vi "LINC Insert Data.vi"(0 "item names":string[](array[string]), 1 "member types":string[](array[string]), 2 "scale":bool, 3 "simulate":bool, 5 "item formats":T1[](array[typedef]), 7 "data in":string, 9 "little endian":bool, 11 "error in (no error)":errorcluster, 12 "member names":string[](array[string]), 13 "member data":string[](array[string])) -> (8 "data out":string, 15 "error out":errorcluster)   [LabVIEW 2018, in "STEPkgDriver_LINC.lvlib"]
uses:
  STEPkgDriver_LINC.lvlib
  LINC Format Prototype.ctl
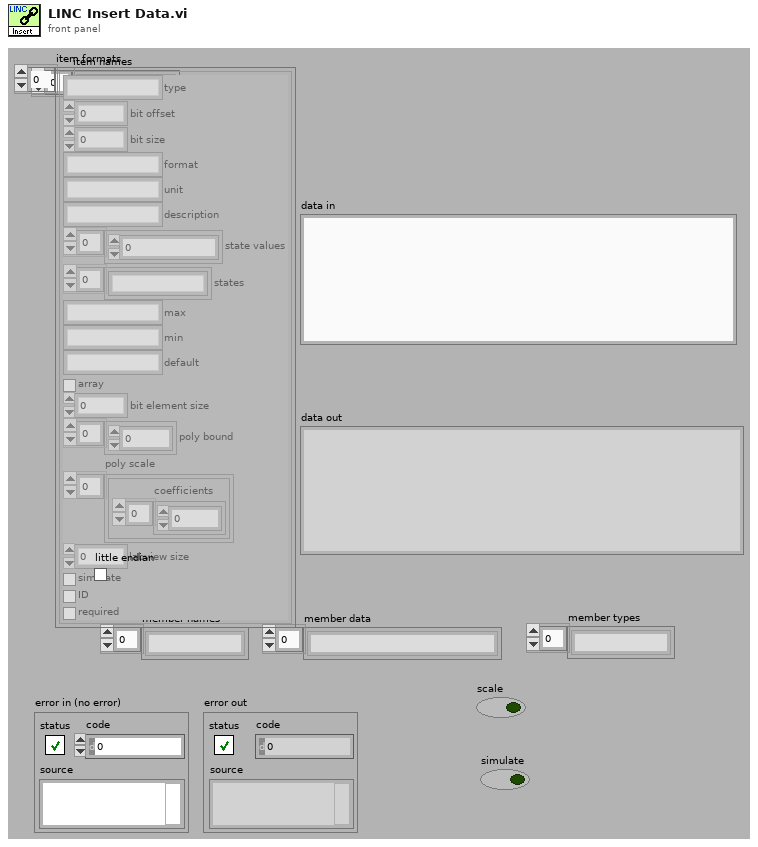
[diagram p1: front panel]
types:
  T1 = typedef "STEPkgDriver_LINC.lvlib/LINC Format Prototype.ctl" = cluster{"type":string, "bit offset":i32, "bit size":i32, "format":string, "unit":string, "description":string, "state values":i64[], "states":string[], "max":string, "min":string, "default":string, "array":bool, "bit element size":i32, "poly bound":dbl[], "poly scale":cluster{"coefficients":dbl[]}[], "labview size":i32, "simulate":bool, "ID":bool, "required":bool}
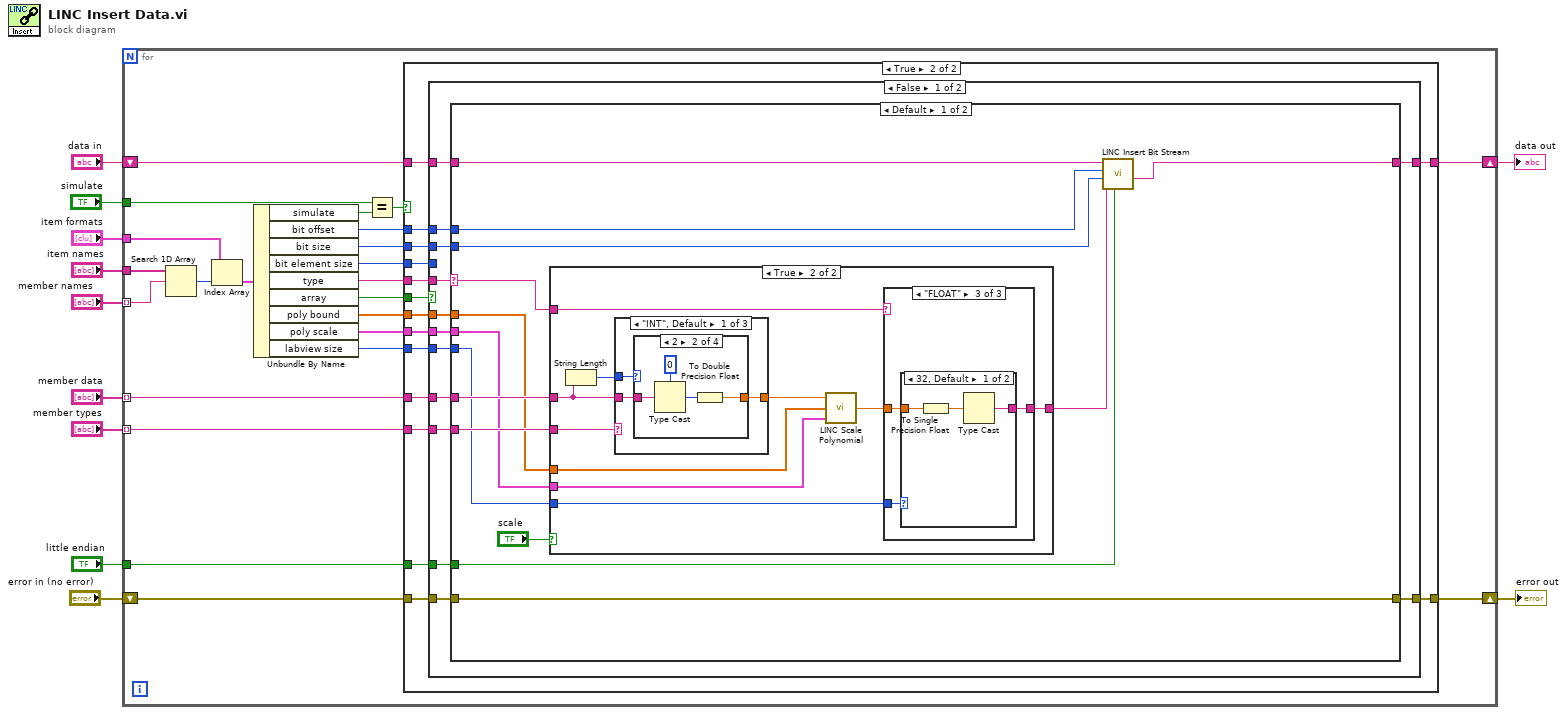
[diagram p0: block diagram]
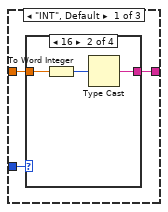
[diagram p4: hidden frame]
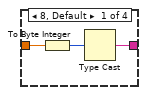
[diagram p5: hidden frame]
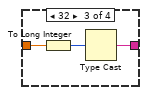
[diagram p6: hidden frame]
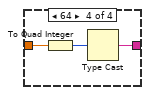
[diagram p7: hidden frame]
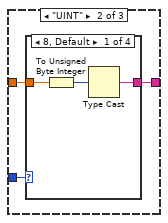
[diagram p8: hidden frame]
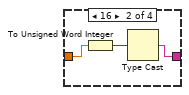
[diagram p9: hidden frame]
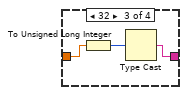
[diagram p10: hidden frame]
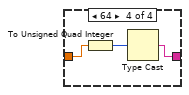
[diagram p11: hidden frame]
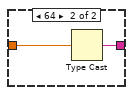
[diagram p12: hidden frame]
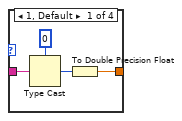
[diagram p13: hidden frame]
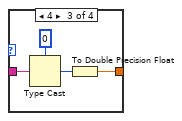
[diagram p14: hidden frame]
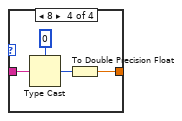
[diagram p15: hidden frame]
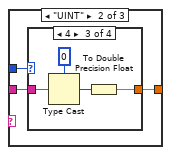
[diagram p16: hidden frame]
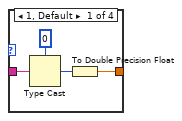
[diagram p17: hidden frame]
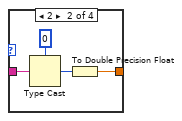
[diagram p18: hidden frame]
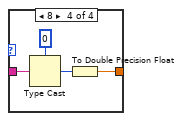
[diagram p19: hidden frame]
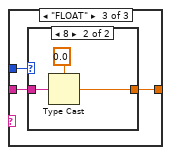
[diagram p20: hidden frame]
diagram:
  n1 = for {
    tunnel: "item formats" -> [w33]
    shift-right: [w23] -> w11
    shift-left: "data in" -> [w26]
    tunnel: "item names" -> [w34]
    tunnel: "member names" -> [w28] mode=indexing
    tunnel: "member data" -> [w27] mode=indexing
    tunnel: "member types" -> [w22] mode=indexing
    tunnel: "simulate" -> [w13]
    tunnel: "little endian" -> [w17]
    shift-right: [w15] -> w1
    shift-left: "error in (no error)" -> [w16]
    n2 = Search 1D Array(1D array=w34, element=w28) -> (index of element=w32:i32)  [unwired: 1 out]
    n3 = Index Array(array=w33, index=w32) -> (element=w31:T1)
    n4 = Unbundle By Name(w31) -> ("simulate"=w14:bool, "bit offset"=w24:i32, "bit size"=w25:i32, "bit element size"=w20:i32, "type"=w30:string, "array"=w29:bool, "poly bound"=w21:dbl[], "poly scale"=w12:cluster{"coefficients":dbl[]}[], "labview size"=w19:i32)
    n5 = Equal?(x=w13, y=w14) -> (x = y?=w18:bool)
    n6 = case shown="True" w18 {
      tunnel: w30 -> [_ w51]
      tunnel: w29 -> [_ w50]
      tunnel: w27 -> [_ w49]
      tunnel: w26 -> [w36 w48]
      tunnel: w25 -> [_ w47]
      tunnel: w24 -> [_ w46]
      tunnel: [w36 w45] -> w23
      tunnel: w22 -> [_ w44]
      tunnel: w21 -> [_ w43]
      tunnel: w20 -> [_ w42]
      tunnel: w19 -> [_ w41]
      tunnel: w17 -> [_ w40]
      tunnel: w16 -> [w35 w39]
      tunnel: [w35 w38] -> w15
      tunnel: w12 -> [_ w37]
      frame False {
      }
      frame True {
        n7 = case shown="False" w50 {
          tunnel: w49 -> [w64 w236]
          tunnel: w51 -> [w63 w235]
          tunnel: [w62 w233] -> w45
          tunnel: w42 -> [_ w223]
          tunnel: w48 -> [w61 w234]
          tunnel: w47 -> [w60 w227]
          tunnel: w46 -> [w59 w230]
          tunnel: w44 -> [w57 _]
          tunnel: w43 -> [w58 _]
          tunnel: w41 -> [w56 _]
          tunnel: w40 -> [w55 w225]
          tunnel: w39 -> [w54 w221]
          tunnel: [w53 w220] -> w38
          tunnel: w37 -> [w52 _]
          frame False {
            n8 = case shown="Default" w63 {
              selector: w63 -> [w75 _]
              tunnel: w64 -> [w77 w179]
              tunnel: [w71 w187] -> w62
              tunnel: w61 -> [w72 w188]
              tunnel: w60 -> [w68 w185]
              tunnel: w59 -> [w69 w183]
              tunnel: w58 -> [w76 _]
              tunnel: w57 -> [w78 _]
              tunnel: w56 -> [w74 _]
              tunnel: w55 -> [w67 _]
              tunnel: w54 -> [w66 w177]
              tunnel: [w66 w176] -> w53
              tunnel: w52 -> [w65 _]
              frame Default {
                n9 = case shown="True" "scale" {
                  tunnel: w78 -> [_ w89]
                  tunnel: w77 -> [w79 w87]
                  tunnel: w76 -> [_ w81]
                  tunnel: w75 -> [_ w86]
                  tunnel: [w79 w85] -> w70
                  tunnel: w74 -> [_ w84]
                  tunnel: w65 -> [_ w80]
                  frame False {
                  }
                  frame True {
                    n10 = String Length(string=w87) -> (length=w88:i32)
                    n11 = case shown="\"INT\", Default" w89 {
                      tunnel: w88 -> [w130 w149 w168]
                      tunnel: w87 -> [w129 w148 w167]
                      tunnel: [w128 w147 w166] -> w83
                      frame "INT", Default {
                        n12 = case shown="2" w130 {
                          tunnel: w129 -> [w134 w138 w142 w146]
                          tunnel: [w131 w135 w139 w143] -> w128
                          frame 1, Default {
                            n13 = Type Cast(type=i8 0, x=w134) -> (*(type *) &x=w133:i8)
                            n14 = To Double Precision Float(number=w133) -> (double precision float=w131:dbl)
                          }
                          frame 2 {
                            n15 = Type Cast(type=i16 0, x=w138) -> (*(type *) &x=w137:i16)
                            n16 = To Double Precision Float(number=w137) -> (double precision float=w135:dbl)
                          }
                          frame 4 {
                            n17 = Type Cast(type=0, x=w142) -> (*(type *) &x=w141:i32)
                            n18 = To Double Precision Float(number=w141) -> (double precision float=w139:dbl)
                          }
                          frame 8 {
                            n19 = Type Cast(type=i64 0, x=w146) -> (*(type *) &x=w145:i64)
                            n20 = To Double Precision Float(number=w145) -> (double precision float=w143:dbl)
                          }
                        }
                      }
                      frame "UINT" {
                        n21 = case shown="4" w149 {
                          tunnel: w148 -> [w153 w157 w161 w165]
                          tunnel: [w150 w154 w158 w162] -> w147
                          frame 1, Default {
                            n22 = Type Cast(type=u8 0, x=w153) -> (*(type *) &x=w152:u8)
                            n23 = To Double Precision Float(number=w152) -> (double precision float=w150:dbl)
                          }
                          frame 2 {
                            n24 = Type Cast(type=u16 0, x=w157) -> (*(type *) &x=w156:u16)
                            n25 = To Double Precision Float(number=w156) -> (double precision float=w154:dbl)
                          }
                          frame 4 {
                            n26 = Type Cast(type=u32 0, x=w161) -> (*(type *) &x=w160:u32)
                            n27 = To Double Precision Float(number=w160) -> (double precision float=w158:dbl)
                          }
                          frame 8 {
                            n28 = Type Cast(type=u64 0, x=w165) -> (*(type *) &x=w164:u64)
                            n29 = To Double Precision Float(number=w164) -> (double precision float=w162:dbl)
                          }
                        }
                      }
                      frame "FLOAT" {
                        n30 = case shown="8" w168 {
                          tunnel: w167 -> [w172 w175]
                          tunnel: [w169 w173] -> w166
                          frame 4, Default {
                            n31 = Type Cast(type=sgl 0.0, x=w172) -> (*(type *) &x=w171:sgl)
                            n32 = To Double Precision Float(number=w171) -> (double precision float=w169:dbl)
                          }
                          frame 8 {
                            n33 = Type Cast(type=0.0, x=w175) -> (*(type *) &x=w173:dbl)
                          }
                        }
                      }
                    }
                    n34 = call "LINC Scale Polynomial.vi"("poly scale"=w80, "poly bounds"=w81, "unscaled value"=w83) -> ("scaled value"=w82:dbl)
                    n35 = case shown="\"FLOAT\"" w86 {
                      tunnel: w82 -> [w92 w107 w122]
                      tunnel: [w91 w106 w121] -> w85
                      tunnel: w84 -> [w90 w105 w120]
                      frame "INT", Default {
                        n36 = case shown="16" w90 {
                          tunnel: w92 -> [w94 w97 w100 w103]
                          tunnel: [w93 w96 w99 w102] -> w91
                          frame 8, Default {
                            n37 = To Byte Integer(number=w94) -> (8bit integer=w95:i8)
                            n38 = Type Cast(x=w95) -> (*(type *) &x=w93:string)  [unwired: 1 in]
                          }
                          frame 16 {
                            n39 = To Word Integer(number=w97) -> (16bit integer=w98:i16)
                            n40 = Type Cast(x=w98) -> (*(type *) &x=w96:string)  [unwired: 1 in]
                          }
                          frame 32 {
                            n41 = To Long Integer(number=w100) -> (32bit integer=w101:i32)
                            n42 = Type Cast(x=w101) -> (*(type *) &x=w99:string)  [unwired: 1 in]
                          }
                          frame 64 {
                            n43 = To Quad Integer(1:w103) -> (0:w104:i64)
                            n44 = Type Cast(x=w104) -> (*(type *) &x=w102:string)  [unwired: 1 in]
                          }
                        }
                      }
                      frame "UINT" {
                        n45 = case shown="8, Default" w105 {
                          tunnel: w107 -> [w109 w112 w115 w118]
                          tunnel: [w108 w111 w114 w117] -> w106
                          frame 8, Default {
                            n46 = To Unsigned Byte Integer(number=w109) -> (unsigned 8bit integer=w110:u8)
                            n47 = Type Cast(x=w110) -> (*(type *) &x=w108:string)  [unwired: 1 in]
                          }
                          frame 16 {
                            n48 = To Unsigned Word Integer(number=w112) -> (unsigned 16bit integer=w113:u16)
                            n49 = Type Cast(x=w113) -> (*(type *) &x=w111:string)  [unwired: 1 in]
                          }
                          frame 32 {
                            n50 = To Unsigned Long Integer(number=w115) -> (unsigned 32bit integer=w116:u32)
                            n51 = Type Cast(x=w116) -> (*(type *) &x=w114:string)  [unwired: 1 in]
                          }
                          frame 64 {
                            n52 = To Unsigned Quad Integer(1:w118) -> (0:w119:u64)
                            n53 = Type Cast(x=w119) -> (*(type *) &x=w117:string)  [unwired: 1 in]
                          }
                        }
                      }
                      frame "FLOAT" {
                        n54 = case shown="32, Default" w120 {
                          tunnel: w122 -> [w124 w126]
                          tunnel: [w123 w127] -> w121
                          frame 32, Default {
                            n55 = To Single Precision Float(number=w124) -> (single precision float=w125:sgl)
                            n56 = Type Cast(x=w125) -> (*(type *) &x=w123:string)  [unwired: 1 in]
                          }
                          frame 64 {
                            n57 = Type Cast(x=w126) -> (*(type *) &x=w127:string)  [unwired: 1 in]
                          }
                        }
                      }
                    }
                  }
                }
                n58 = call "LINC Insert Bit Stream.vi"("little endian"=w67, "data to insert"=w70, "bit size"=w68, "bit offset"=w69, "data in"=w72) -> ("data out"=w71:string)  [unwired: 4 in]
              }
              frame "BLOCK", "STRING" {
                n59 = Unflatten From String(type="", binary string=w179) -> (value=w178:string)  [unwired: 3 in, 2 out]
                n60 = Quotient & Remainder(x=w183, y=8) -> (floor(x/y)=w182:i32)  [unwired: 1 out]
                n61 = Quotient & Remainder(x=w185, y=8) -> (floor(x/y)=w181:i32)  [unwired: 1 out]
                n62 = case shown="..0" w181 {
                  selector: w181 -> [_ w196]
                  tunnel: w188 -> [w195 w206]
                  tunnel: [w190 w205] -> w187
                  tunnel: w182 -> [w194 w204]
                  tunnel: w178 -> [w191 w203]
                  tunnel: w177 -> [w189 w201]
                  tunnel: [w189 w198] -> w176
                  frame ..0 {
                    n63 = String Subset(string=w195, offset (0)=0, length (rest)=w194) -> (substring=w192:string)
                    n64 = Concatenate Strings(w192, w191) -> (w190:string)
                  }
                  frame 1.. {
                    n65 = Initialize Array(u8 0, w196) -> (w208:u8[])
                    n66 = Byte Array To String(unsigned byte array=w208) -> (string=w207:string)
                    n67 = Replace Substring(4:w203, 5:w207) -> (1:w199:string)  [unwired: 3 out]
                    n68 = String Length(string=w199) -> (length=w202:i32)
                    n69 = Greater?(x=w202, y=w196) -> (0:w200:bool)
                    n70 = case shown="True" w200 {
                      tunnel: w201 -> [w210 w215]
                      tunnel: w199 -> [w211 w219]
                      tunnel: [w211 w216] -> w197
                      tunnel: [w210 w214] -> w198
                      tunnel: w196 -> [_ w217]
                      frame False {
                      }
                      frame True {
                        n71 = String Subset(string=w219, offset (0)=0, length (rest)=w217) -> (substring=w216:string)
                        n72 = call "Generate Error.vi"("error code (-1301)"=9099, "error in"=w215, "description"="String or Block passed is larger than defined.") -> ("error out"=w214:errorcluster)  [unwired: 8 in]
                      }
                    }
                    n73 = Replace Substring(3:w204, 4:w197, 5:w206) -> (1:w205:string)  [unwired: 2 out]
                  }
                }
              }
            }
          }
          frame True {
            n74 = Quotient & Remainder(x=w230, y=8) -> (floor(x/y)=w229:i32)  [unwired: 1 out]
            n75 = Quotient & Remainder(x=w227, y=8) -> (floor(x/y)=w226:i32)  [unwired: 1 out]
            n76 = Quotient & Remainder(x=w223, y=8) -> (floor(x/y)=w222:i32)  [unwired: 1 out]
            n77 = case shown="\"BLOCK\", \"STRING\"" w235 {
              tunnel: w236 -> [w247 w269]
              tunnel: [w243 w266] -> w232
              tunnel: w226 -> [w238 w267]
              tunnel: w225 -> [w242 _]
              tunnel: w222 -> [w239 w268]
              tunnel: w221 -> [w237 w265]
              tunnel: [w237 w264] -> w220
              frame Default {
                # "remove size"
                n78 = String Subset(string=w247, offset (0)=4) -> (substring=w241:string)  [unwired: 1 in]
                n79 = Initialize Array(u8 0, w238) -> (w245:u8[])
                n80 = Byte Array To String(unsigned byte array=w245) -> (string=w244:string)
                n81 = case shown="True" w242 {
                  tunnel: w241 -> [w249 w253]
                  tunnel: [w249 w252] -> w240
                  tunnel: w239 -> [_ w251]
                  tunnel: w238 -> [_ w250]
                  frame False {
                  }
                  frame True {
                    n82 = Quotient & Remainder(x=w250, y=w251) -> (floor(x/y)=w254:i32)  [unwired: 1 out]
                    n83 = for {
                      N: w254 -> [_]
                      shift-right: [w258] -> w252
                      shift-left: w253 -> [w259]
                      shift-right: [w262] -> _
                      shift-left: 0 -> [w256]
                      tunnel: w251 -> [w263]
                      tunnel: w251 -> [w261]
                      n84 = String Subset(string=w259, offset (0)=w256, length (rest)=w263) -> (substring=w260:string)
                      n85 = Add(x=w256, y=w261) -> (x+y=w262:i32)
                      n86 = Reverse String(1:w260) -> (0:w257:string)
                      n87 = Replace Substring(3:w256, 4:w257, 5:w259) -> (1:w258:string)  [unwired: 1 in, 1 out]
                    }
                  }
                }
                n88 = Replace Substring(4:w240, 5:w244) -> (1:w243:string)  [unwired: 3 out]
              }
              frame "BLOCK", "STRING" {
                n89 = Initialize Array(u8 0, w267) -> (w271:u8[])
                n90 = Unflatten From String(type=string[] [], binary string=w269) -> (value=w273:string[])  [unwired: 3 in, 2 out]
                n91 = Byte Array To String(unsigned byte array=w271) -> (string=w275:string)
                n92 = for {
                  shift-right: [w285] -> w266
                  shift-left: w275 -> [w286]
                  tunnel: w273 -> [w277] mode=indexing
                  shift-right: [w284] -> _
                  shift-left: 0 -> [w283]
                  tunnel: w268 -> [w276]
                  shift-right: [w278] -> w264
                  shift-left: w265 -> [w279]
                  n93 = String Length(string=w277) -> (length=w281:i32)
                  n94 = Greater?(x=w281, y=w276) -> (0:w280:bool)
                  n95 = String Subset(string=w277, length (rest)=w276) -> (substring=w282:string)  [unwired: 1 in]
                  n96 = case shown="True" w280 {
                    tunnel: w279 -> [w287 w291]
                    tunnel: [w287 w290] -> w278
                    frame False {
                    }
                    frame True {
                      n97 = call "Generate Error.vi"("error code (-1301)"=9099, "error in"=w291, "description"="String or Block passed is larger than defined.") -> ("error out"=w290:errorcluster)  [unwired: 8 in]
                    }
                  }
                  n98 = Add(x=w283, y=w276) -> (x+y=w284:i32)
                  n99 = Replace Substring(3:w283, 4:w282, 5:w286) -> (1:w285:string)  [unwired: 2 out]
                }
              }
            }
            n100 = Replace Substring(3:w229, 4:w232, 5:w234) -> (1:w233:string)  [unwired: 2 out]
          }
        }
      }
    }
  }
  "data out" <- w11
  "error out" <- w1
